vi "Next Generation.vi"(8 "error in":errorcluster, 11 "cells in":bool[][](array[boolean])=[[FALSE, FALSE, TRUE, FALSE, FALSE, FALSE, FALSE, FALSE, FALSE, FALSE, FALSE, FALSE, FALSE, FALSE, FALSE, FALSE], [FALSE, FALSE, FALSE, TRUE, TRUE, FALSE, FALSE, FALSE, FALSE, FALSE, FALSE, FALSE, FALSE, FALSE, FALSE, FALSE], [FALSE, FALSE, FALSE, FALSE, FALSE, FALSE, FALSE, FALSE, FALSE, FALSE, FALSE, FALSE, FALSE, FALSE, FALSE, FALSE], [FALSE, FALSE, FALSE, FALSE, FALSE, FALSE, FALSE, FALSE, FALSE, FALSE, FALSE, FALSE, FALSE, FALSE, FALSE, FALSE], [FALSE, FALSE, FALSE, FALSE, FALSE, FALSE, FALSE, FALSE, FALSE, FALSE, FALSE, FALSE, FALSE, FALSE, FALSE, FALSE], [FALSE, FALSE, FALSE, FALSE, FALSE, FALSE, FALSE, FALSE, FALSE, FALSE, FALSE, FALSE, FALSE, FALSE, FALSE, FALSE], [FALSE, FALSE, FALSE, FALSE, FALSE, FALSE, FALSE, TRUE, FALSE, FALSE, FALSE, FALSE, FALSE, FALSE, FALSE, FALSE], [FALSE, FALSE, FALSE, FALSE, FALSE, FALSE, FALSE, FALSE, FALSE, FALSE, FALSE, FALSE, FALSE, FALSE, FALSE, FALSE], [FALSE, FALSE, FALSE, FALSE, FALSE, FALSE, FALSE, FALSE, FALSE, FALSE, FALSE, FALSE, FALSE, FALSE, FALSE, FALSE], [FALSE, FALSE, FALSE, FALSE, FALSE, FALSE, FALSE, FALSE, FALSE, FALSE, FALSE, FALSE, FALSE, TRUE, FALSE, FALSE], [FALSE, FALSE, FALSE, FALSE, FALSE, FALSE, FALSE, FALSE, FALSE, FALSE, FALSE, FALSE, TRUE, TRUE, FALSE, FALSE], [FALSE, FALSE, FALSE, FALSE, FALSE, FALSE, FALSE, FALSE, FALSE, FALSE, FALSE, FALSE, FALSE, FALSE, TRUE, FALSE], [FALSE, FALSE, FALSE, FALSE, FALSE, FALSE, FALSE, FALSE, FALSE, FALSE, FALSE, FALSE, FALSE, FALSE, FALSE, TRUE]]) -> (0 "error out":errorcluster, 1 "deaths":i32, 2 "births":i32, 3 "cells out":bool[][](array[boolean])=[[FALSE, FALSE, FALSE, TRUE, FALSE, FALSE, FALSE, FALSE, FALSE, FALSE, FALSE, FALSE, FALSE, FALSE, FALSE, FALSE], [FALSE, FALSE, FALSE, TRUE, FALSE, FALSE, FALSE, FALSE, FALSE, FALSE, FALSE, FALSE, FALSE, FALSE, FALSE, FALSE], [FALSE, FALSE, FALSE, FALSE, FALSE, FALSE, FALSE, FALSE, FALSE, FALSE, FALSE, FALSE, FALSE, FALSE, FALSE, FALSE], [FALSE, FALSE, FALSE, FALSE, FALSE, FALSE, FALSE, FALSE, FALSE, FALSE, FALSE, FALSE, FALSE, FALSE, FALSE, FALSE], [FALSE, FALSE, FALSE, FALSE, FALSE, FALSE, FALSE, FALSE, FALSE, FALSE, FALSE, FALSE, FALSE, FALSE, FALSE, FALSE], [FALSE, FALSE, FALSE, FALSE, FALSE, FALSE, FALSE, FALSE, FALSE, FALSE, FALSE, FALSE, FALSE, FALSE, FALSE, FALSE], [FALSE, FALSE, FALSE, FALSE, FALSE, FALSE, FALSE, FALSE, FALSE, FALSE, FALSE, FALSE, FALSE, FALSE, FALSE, FALSE], [FALSE, FALSE, FALSE, FALSE, FALSE, FALSE, FALSE, FALSE, FALSE, FALSE, FALSE, FALSE, FALSE, FALSE, FALSE, FALSE], [FALSE, FALSE, FALSE, FALSE, FALSE, FALSE, FALSE, FALSE, FALSE, FALSE, FALSE, FALSE, FALSE, FALSE, FALSE, FALSE], [FALSE, FALSE, FALSE, FALSE, FALSE, FALSE, FALSE, FALSE, FALSE, FALSE, FALSE, FALSE, TRUE, TRUE, FALSE, FALSE], [FALSE, FALSE, FALSE, FALSE, FALSE, FALSE, FALSE, FALSE, FALSE, FALSE, FALSE, FALSE, TRUE, TRUE, TRUE, FALSE], [FALSE, FALSE, FALSE, FALSE, FALSE, FALSE, FALSE, FALSE, FALSE, FALSE, FALSE, FALSE, FALSE, TRUE, TRUE, FALSE], [FALSE, FALSE, FALSE, FALSE, FALSE, FALSE, FALSE, FALSE, FALSE, FALSE, FALSE, FALSE, FALSE, FALSE, FALSE, FALSE]])   [LabVIEW 2021, in "Game of Life.lvlib"]
doc: "Any live cell with two or three live neighbors lives on to the next generation. Any dead cell with exactly three live neighbors becomes a live cell, as if by reproduction."
uses:
  Game of Life.lvlib
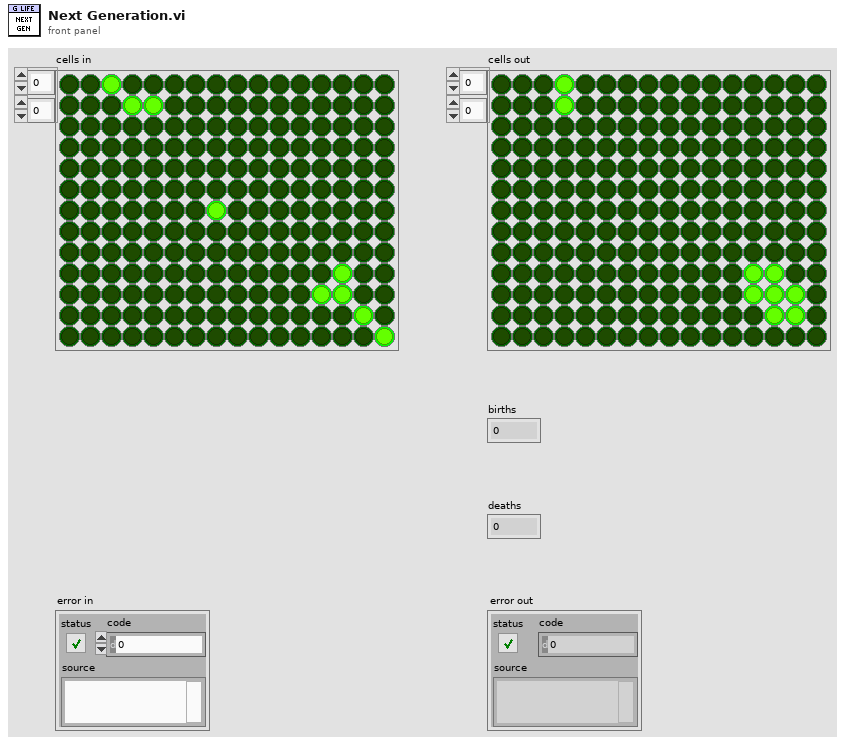
[diagram p1: front panel]
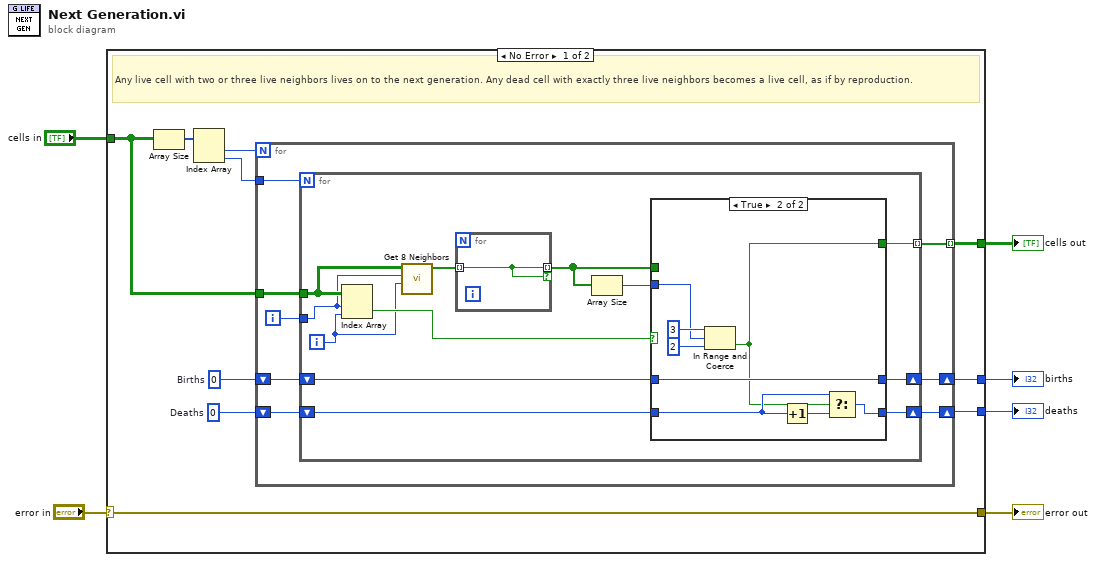
[diagram p0: block diagram]
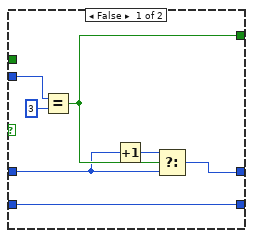
[diagram p2: hidden frame]
diagram:
  n1 = case shown="No Error" "error in" {
    selector: "error in" -> [w7 w54]
    tunnel: [w13 _] -> w6
    tunnel: [w10 _] -> w5
    tunnel: "cells in" -> [w9 w53]
    tunnel: [w8 w53] -> w3
    tunnel: [w7 w54] -> w1
    frame No Error {
      w11 = 0  # Deaths
      w12 = 0  # Births
      # "Any live cell with two or three live neighbors lives on to the next generation. Any dead cell with exactly three live neighbors becomes a live cell, as if by reproduction."
      n2 = Array Size(array=w9) -> (size(s)=w16:i32[])
      n3 = Index Array(array=w16) -> (element #1=w15:i32, element #2=w14:i32)  [unwired: 2 in]
      n4 = for {
        N: w15 -> [_]
        tunnel: w14 -> [w23]
        tunnel: [w22] -> w8 mode=indexing
        shift-right: [w21] -> w13
        shift-left: w12 -> [w20]
        shift-right: [w18] -> w10
        shift-left: w11 -> [w19]
        tunnel: w9 -> [w17]
        i -> [w24]
        n5 = for {
          N: w23 -> [_]
          tunnel: w24 -> [w29]
          tunnel: [w36] -> w22 mode=indexing
          shift-right: [w35] -> w21
          shift-left: w20 -> [w34]
          shift-right: [w32] -> w18
          shift-left: w19 -> [w33]
          tunnel: w17 -> [w30]
          i -> [w28]
          n6 = Index Array(array=w30, index (row)=w29, index (col)=w28) -> (element=w31:bool)
          n7 = call "Get 8 Neighbors.vi"("column"=w28, "row"=w29, "cells in"=w30) -> ("cells living"=w27:bool[])  [unwired: 8 in]
          n8 = for {
            tunnel: w27 -> [w37] mode=indexing
            tunnel: [w37] -> w25 mode=indexing if=w37
          }
          n9 = Array Size(array=w25) -> (size(s)=w26:i32)
          n10 = case shown="True" w31 {
            tunnel: [w42 w46] -> w36
            tunnel: [w39 w50] -> w35
            tunnel: w34 -> [w38 w50]
            tunnel: w33 -> [w40 w48]
            tunnel: [w40 w45] -> w32
            tunnel: w26 -> [w43 w49]
            tunnel: w25 -> [_ _]
            frame False {
              n11 = Equal?(x=w43, y=3) -> (x = y?=w42:bool)
              n12 = Increment(x=w38) -> (x+1=w41:i32)
              n13 = Select(t=w41, s=w42, f=w38) -> (s? t:f=w39:i32)
            }
            frame True {
              n14 = In Range and Coerce(upper limit=3, x=w49, lower limit=2) -> (In Range?=w46:bool)  [unwired: 1 out]
              n15 = Increment(x=w48) -> (x+1=w47:i32)
              n16 = Select(t=w48, s=w46, f=w47) -> (s? t:f=w45:i32)
            }
          }
        }
      }
    }
    frame Error {
    }
  }
  "births" <- w6
  "deaths" <- w5
  "cells out" <- w3
  "error out" <- w1
